vi "_attribute_read_rawstring.vi"(5 "Repeated Capability":string, 7 "Attribute":T1={"Identifier"="", "Descriptive Name"="", "Data Type"=enum."Integer 32", "Command"="", "Access"=enum."Read/Write", "Range Table"="", "Read Callback"="", "Write Callback"="", "Supported Models"="", "Instrument Options"="", "Index"=0, "OPC Wait"=FALSE, "No Status Check"=FALSE, "Cache Only"=FALSE}, 8 "error in":errorcluster caption="error in (no error)", 10 "Query Parameter":string, 11 "VISA resource name":refnum<visa-resource-name>) -> (0 "error out":errorcluster, 2 "String out":string, 3 "VISA resource name out":refnum<visa-resource-name>)   [LabVIEW 2022 SP3, in "hmp4000_rsidr_core.lvlib"]
uses:
  hmp4000_rsidr_core.lvlib
  type_Attribute.ctl
  type_Attribute_Data_Type.ctl
  type_ReadWriteAccess.ctl
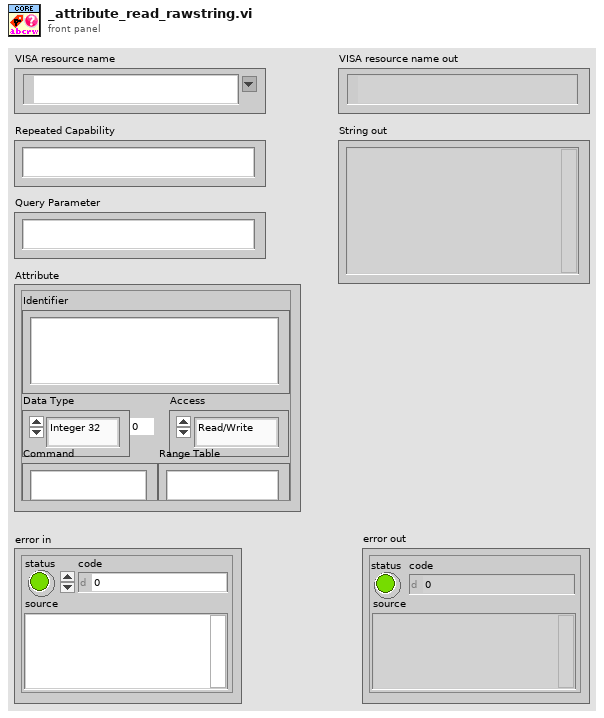
[diagram p1: front panel]
types:
  T1 = typedef "hmp4000_rsidr_core.lvlib/type_Attribute.ctl" = cluster{"Identifier":string, "Descriptive Name":string, "Data Type":T2, "Command":string, "Access":T3, "Range Table":string, "Read Callback":string, "Write Callback":string, "Supported Models":string, "Instrument Options":string, "Index":i32, "OPC Wait":bool, "No Status Check":bool, "Cache Only":bool}
  T2 = typedef "hmp4000_rsidr_core.lvlib/type_Attribute_Data_Type.ctl" = enum16{"Integer 32", "Double", "String", "Boolean", "None", "Integer 64", "RawString"}
  T3 = typedef "hmp4000_rsidr_core.lvlib/type_ReadWriteAccess.ctl" = enum16{"Read Only", "Write Only", "Read/Write"}
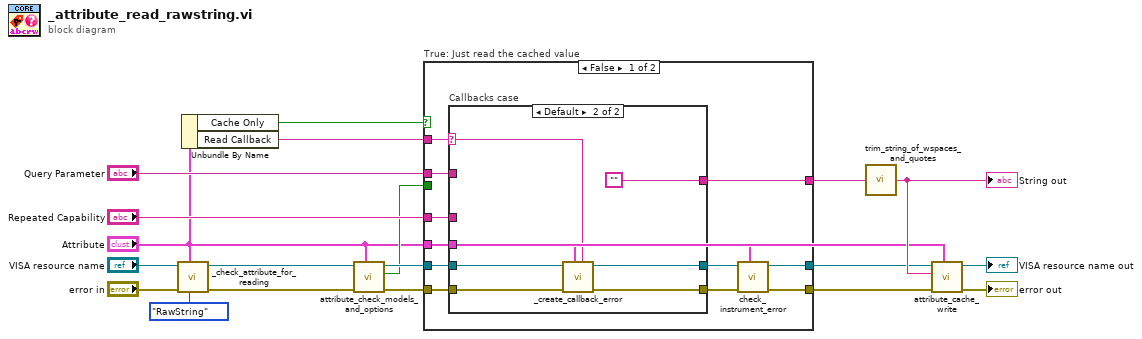
[diagram p0: block diagram]
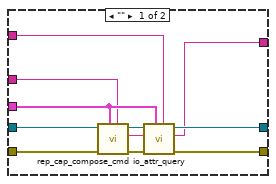
[diagram p2: hidden frame]
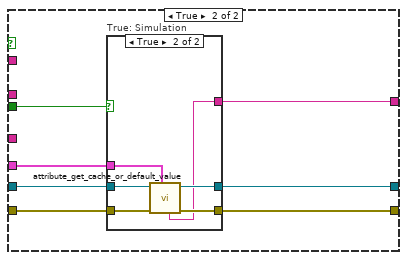
[diagram p3: hidden frame]
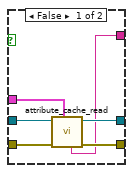
[diagram p4: hidden frame]
diagram:
  n1 = call "_check_attribute_for_reading.vi"("Expected Data Type"=type_Attribute_Data_Type."RawString" ("Data Type"), "Attribute"="Attribute", "error in"="error in", "VISA resource name"="VISA resource name") -> ("error out"=w7:errorcluster, "VISA resource name out"=w6:refnum<visa-resource-name>)  [unwired: 6 in]
  n2 = Unbundle By Name("Attribute") -> ("Cache Only"=w1:bool, "Read Callback"=w10:string)
  n3 = call "attribute_check_models_and_options.vi"("Attribute"="Attribute", "error in"=w7, "VISA resource name"=w6) -> ("error out"=w5:errorcluster, "Simulation Mode"=w3:bool, "VISA resource name out"=w4:refnum<visa-resource-name>)  [unwired: 6 in]
  n4 = case "True: Just read the cached value" shown="False" w1 {
    tunnel: "Repeated Capability" -> [w30 _]
    tunnel: [w22 w51] -> w9
    tunnel: [w21 w52] -> w8
    tunnel: [w29 w50] -> w13
    tunnel: w10 -> [w28 _]
    tunnel: w4 -> [w27 w55]
    tunnel: w5 -> [w26 w53]
    tunnel: "Attribute" -> [w20 w54]
    tunnel: w3 -> [_ w49]
    tunnel: "Query Parameter" -> [w25 _]
    frame False {
      n5 = case "Callbacks case" shown="Default" w28 {
        selector: w28 -> [_ w44]
        tunnel: w27 -> [w41 w47]
        tunnel: w26 -> [w40 w48]
        tunnel: w30 -> [w33 _]
        tunnel: [w39 w45] -> w23
        tunnel: [w38 w46] -> w24
        tunnel: [w32 "" ("Empty String Constant")] -> w29
        tunnel: w20 -> [w34 w43]
        tunnel: w25 -> [w31 _]
        frame "" {
          n6 = call "rep_cap_compose_cmd.vi"("Repeated Capability"=w33, "Attribute"=w34, "error in"=w40, "VISA resource name"=w41) -> ("error out"=w37:errorcluster, "Command out"=w36:string, "VISA resource name out"=w35:refnum<visa-resource-name>)  [unwired: 5 in]
          n7 = call "io_attr_query.vi"("Query Parameter (None)"=w31, "Attribute"=w34, "error in"=w37, "write buffer"=w36, "VISA resource name"=w35) -> ("error out"=w38:errorcluster, "read buffer"=w32:string, "VISA resource name out"=w39:refnum<visa-resource-name>)  [unwired: 4 in]
        }
        frame Default {
          n8 = call "_create_callback_error.vi"("Callback Name"=w44, "Attribute"=w43, "error in"=w48, "VISA resource name"=w47) -> ("error out"=w46:errorcluster, "VISA resource name out"=w45:refnum<visa-resource-name>)  [unwired: 6 in]
        }
      }
      n9 = call "check_instrument_error.vi"("Attribute"=w20, "error in"=w24, "VISA resource name"=w23) -> ("error out"=w22:errorcluster, "VISA resource name out"=w21:refnum<visa-resource-name>)  [unwired: 7 in]
    }
    frame True {
      n10 = case "True: Simulation" shown="True" w49 {
        tunnel: w53 -> [w61 w67]
        tunnel: w55 -> [w60 w66]
        tunnel: w54 -> [w59 w63]
        tunnel: [w58 w65] -> w51
        tunnel: [w57 w64] -> w52
        tunnel: [w56 w62] -> w50
        frame False {
          n11 = call "attribute_cache_read.vi"("Attribute"=w59, "error in"=w61, "VISA resource name"=w60) -> ("error out"=w58:errorcluster, "VISA resource name out"=w57:refnum<visa-resource-name>, "String out"=w56:string)  [unwired: 1 in, 5 out]
        }
        frame True {
          n12 = call "attribute_get_cache_or_default_value.vi"("Attribute"=w63, "error in"=w67, "VISA resource name"=w66) -> ("error out"=w65:errorcluster, "VISA resource name out"=w64:refnum<visa-resource-name>, "String out"=w62:string)  [unwired: 1 in, 5 out]
        }
      }
    }
  }
  n13 = call "trim_string_of_wspaces_and_quotes.vi"("String in"=w13) -> ("String out"=w12:string)  [unwired: 4 in]
  "String out" <- w12
  n14 = call "attribute_cache_write.vi"("Attribute"="Attribute", "error in"=w9, "Value in"=w12, "VISA resource name"=w8) -> ("error out"=→"error out":errorcluster, "VISA resource name out"=→"VISA resource name out":refnum<visa-resource-name>)  [unwired: 6 in]
